vi "ReadDeviceSpreadsheet.vi"() -> ()   [LabVIEW 2017]
uses:
  <vilib>/addons/_office/excel.llb/Excel Get Data ([str]).vi
  <vilib>/Utility/NIReport.llb/NI_report.lvclass
  <vilib>/addons/_office/NI_ReportGenerationToolkit.lvlib
  <vilib>/Utility/NIReport.llb/Excel/NI_Excel.lvclass
panel:
  out "WorkSheet":string[][](array[string])
  out "Error Out":errorcluster
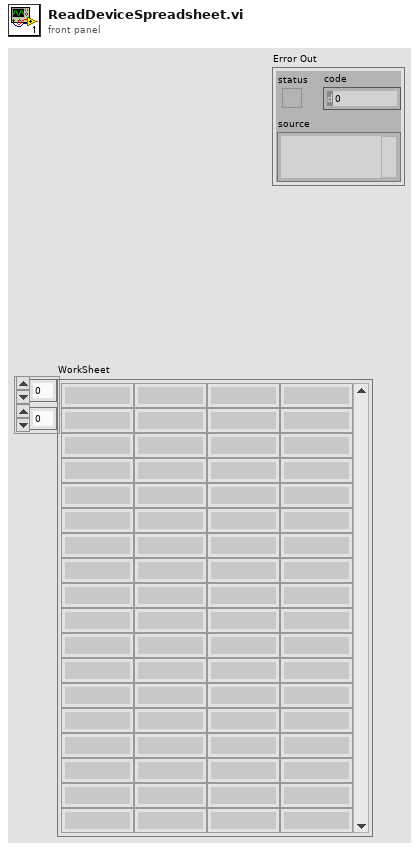
[diagram p1: front panel]
types:
  T1 = enum16{"Standard Report", "HTML", "Word", "Excel"}
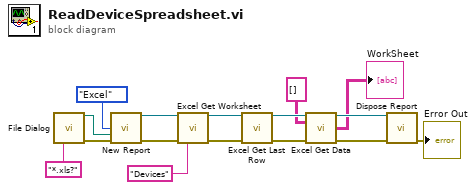
[diagram p0: block diagram]
diagram:
  n1 = call "File Dialog"("pattern (all files)"="*.xls?") -> ("selected path"=w14:path, "error out"=w15:errorcluster)  [unwired: 11 in, 2 out]
  n2 = call <vilib>:"New Report.vi"("report type"=T1."Excel", "template (empty)"=w14, "error in (no error)"=w15) -> ("report out"=w11:refnum<class "NI_report.lvclass">, "error out"=w12:errorcluster)  [unwired: 11 in]
  n3 = call <vilib>:"Excel Get Worksheet.vi"("report in"=w11, "error in (no error)"=w12, "name (\"\")"="Devices" ("name (\"\")")) -> ("report out"=w9:refnum<class "NI_report.lvclass">, "error out"=w10:errorcluster)  [unwired: 11 in]
  n4 = call <vilib>:"Excel Get Last Row.vi"("report in"=w9, "error in (no error)"=w10) -> ("report out"=w8:refnum<class "NI_report.lvclass">, "error out"=w7:errorcluster)  [unwired: 11 in, 1 out]
  n5 = call-poly <vilib>:"Excel Get Data.vi"("report in"=w8, "data type"=string[][] [], "error in (no error)"=w7) -> ("report out"=w4:refnum<class "NI_report.lvclass">, "data"=→"WorkSheet":string[][], "error out"=w5:errorcluster)  [unwired: 10 in]
  n6 = call-dynamic "Dispose Report.vi"("report in"=w4, "error in (no error)"=w5) -> ("error out"=→"Error Out":errorcluster)  [unwired: 13 in]
